vi "4. SJCubeRunExp.vi"() -> ()   [LabVIEW 2019, in "SJCube.lvlib"]
uses:
  SJCube.lvlib
  PendulumState.ctl
  <vilib>/Platform/TimedLoop/XDataNode/timing_clust.ctl
  <vilib>/Platform/TimedLoop/XDataNode/nitl_modes.ctl
  <vilib>/Platform/TimedLoop/XDataNode/wakeup.ctl
  <vilib>/myRIO/Common/Instrument Driver Framework/myRIO v1.0/UART/vis/myRIO v1.0 Close UART.vi
  <vilib>/addons/control/pid/pid.llb/PID (DBL).vi
  <vilib>/myRIO/Common/Instrument Driver Framework/Utilities/vis/FPGA Ref Manager.vi
  <vilib>/myRIO/Common/Instrument Driver Framework/myRIO v1.0/myRIO v1.0 Reset FPGA.vi
  <vilib>/myRIO/Common/Instrument Driver Framework/myRIO v1.0/IRQ/vis/myRIO v1.0 IRQ Info FGV.vi
  <vilib>/myRIO/Common/Instrument Driver Framework/myRIO v1.0/IRQ/vis/myRIO v1.0 Timer IRQ Info FGV.vi
  <vilib>/myRIO/Common/Instrument Driver Framework/myRIO v1.0/IRQ/vis/myRIO v1.0 ISR Agent.vi
  <vilib>/myRIO/Instrument Drivers/Utilities/vis/Reset Index.vi
  <vilib>/myRIO/Common/Instrument Driver Framework/myRIO v1.0/Resource Manager/vis/myRIO v1.0 Block Write Resource Manager.vi
  <vilib>/Platform/TimedLoop/XDataNode/XDataNode.xnode
  <vilib>/Platform/TimedLoop/XDataNode/XDNodeRunTimeDep.lvlib
  <vilib>/myRIO/Instrument Drivers/Utilities/Utilities.lvlib
  <vilib>/addons/control/pid/NI_PID_pid.lvlib
  KNRmBalanceStick-Program/KNRm_ReMi_OS5.lvlibp
  KNRmBalanceStick-Program/KNRm_ReMi_OS5.lvlibp/KNRm_ReMi_Toolkit/IO/LowLevel/IO_Channel_DIO.ctl
panel:
  in  "StickPosControl":bool=TRUE
  out "touch":bool
  in  "Auto\nSetpoint":bool
  out "LATE":bool
  out "停滯":bool
  out "方向":bool
  out "Array":T1[](array[typedef])
  in  "motorPID":T2={"proportional gain (Kc)"=5.0, "integral time (Ti, min)"=0.0, "derivative time (Td, min)"=0.0005}
  in  "PosPID":T2={"proportional gain (Kc)"=-0.05999999999999999, "integral time (Ti, min)"=0.03, "derivative time (Td, min)"=0.019999999999999997}
  in  "BalancePID":T2={"proportional gain (Kc)"=0.07999999999999999, "integral time (Ti, min)"=0.0, "derivative time (Td, min)"=0.0008}
  out "nowState":T1
  out "Waveform Chart":T3(graph)
  in  "Setpoint(deg)":dbl(knob) scale=80.0..-80.0
  out "error out":errorcluster
  out "Position(deg)":dbl(knob) scale=80.0..-80.0
  in  "Reset":bool
  in  "Stop Button":bool
  out "MotorResetPOS":dbl[](array[numeric])
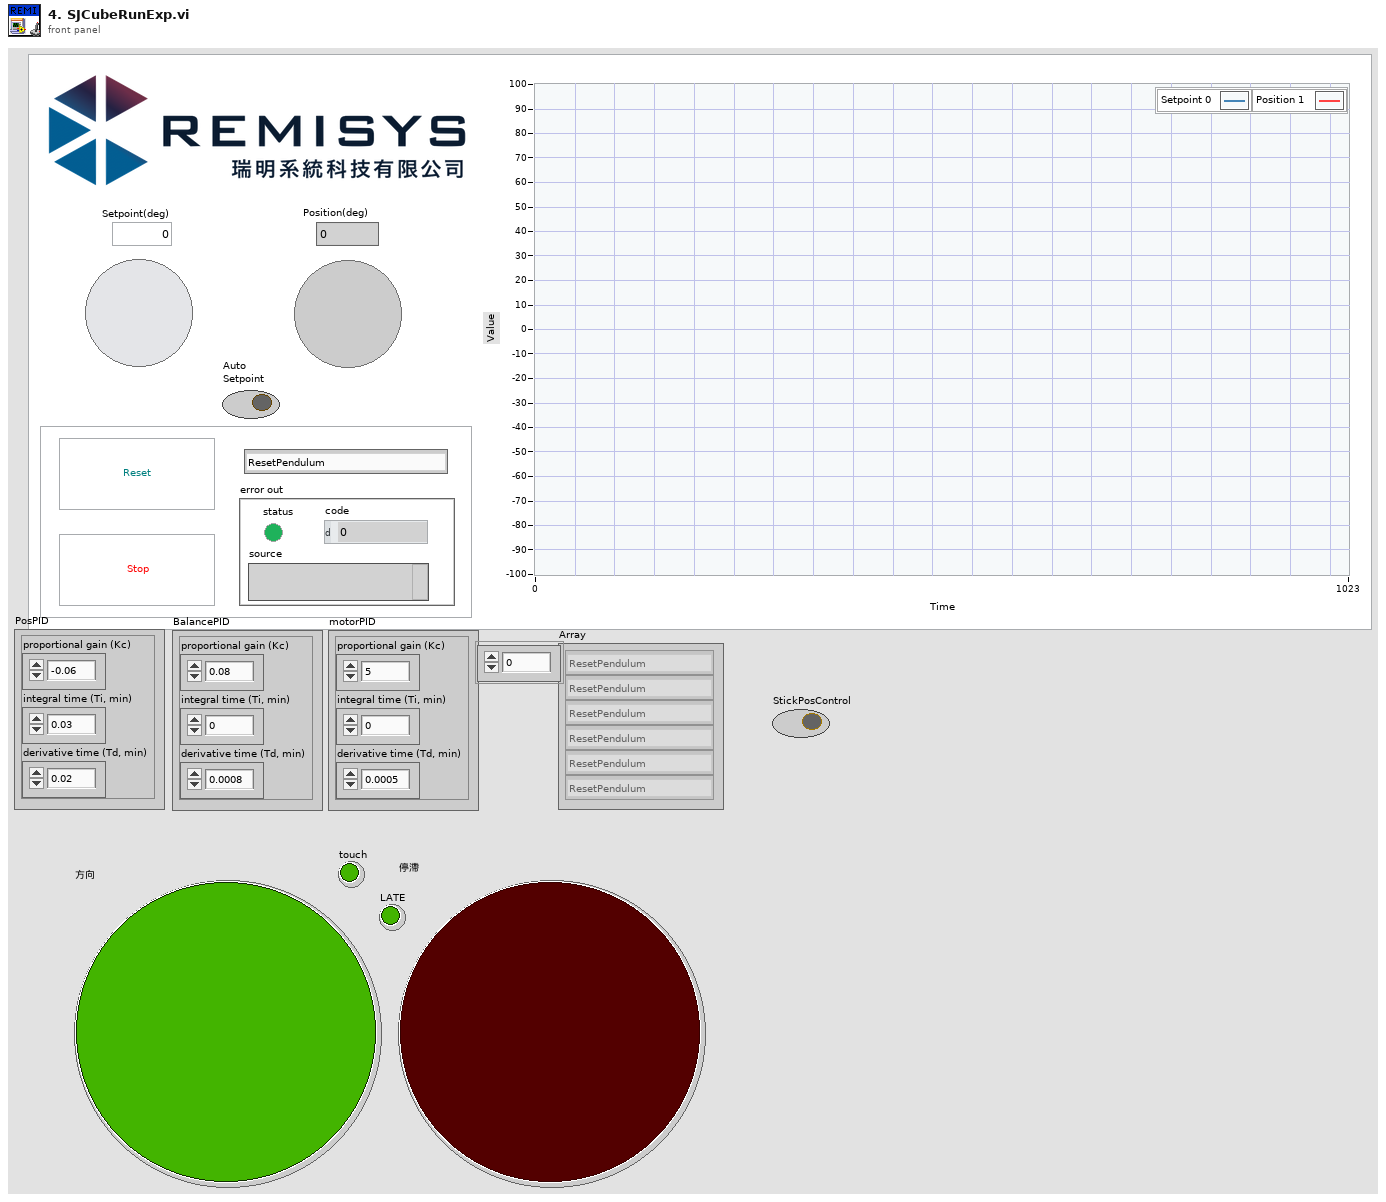
[diagram p1: front panel]
types:
  T1 = typedef "SJCube.lvlib/PendulumState.ctl" = enum16{"ResetPendulum", "PendulumFindHome", "PendulumToHome", "SwingUp", "Balancing", "ExitExp."}
  T2 = cluster{"proportional gain (Kc)":dbl, "integral time (Ti, min)":dbl, "derivative time (Td, min)":dbl}
  T3 = cluster{"Setpoint(deg)":dbl, "PresentPOS(deg)":dbl}
  T4 = typedef "KNRm_ReMi_OS5.lvlibp/IO_Channel_DIO.ctl" = enum16{"B/DIO1 (M1)", "A/DIO8 (M2)", "B/DIO7 (M3)", "A/DIO3 (M4)", "A/DIO14 (RC1_0)", "A/DIO15 (RC1_1)"}
  T5 = typedef "XDNodeRunTimeDep.lvlib/timing_clust.ctl" = cluster{"Expected End [f-1]":u64, "Actual End [f-1]":u64, "Finished Late? [f-1]":bool, "Expected End [i-1]":u64, "Actual End [i-1]":u64, "Finished Late? [i-1]":bool, "Expected Start [i]":u64, "Actual Start [i]":u64, "Expected Start [f]":u64, "Actual Start [f]":u64, "Source Name":string, "Structure Name":string, "Period":i64, "Deadline":i64, "Offset":i64, "Start":i64, "Priority":i32, "Timeout":i32, "Mode":T6, "Wakeup Reason":T7, "Error":errorcluster, "Source Type":string, "Secondary Source Type":string, "Global End Time":u64, "Global Start Time":u64, "Frame Duration":u64, "Iteration Duration":u64, "Assigned CPU":i32, "I/O Scan Engine Mode":u32}
  T6 = typedef "XDNodeRunTimeDep.lvlib/nitl_modes.ctl" = enum32{"No Change", "Process missed periods, maintain original phase", "Discard missed periods, maintain original phase", "Process missed periods, ignore original phase", "Discard missed periods, ignore original phase"}
  T7 = typedef "XDNodeRunTimeDep.lvlib/wakeup.ctl" = enum32{"Normal", "Aborted", "Asynchronous wakeup", "Timing source error", "Timed loop error", "Timeout"}
  T8 = cluster{"Setpoint(deg)":dbl, "MotorEncoder (deg)":dbl}
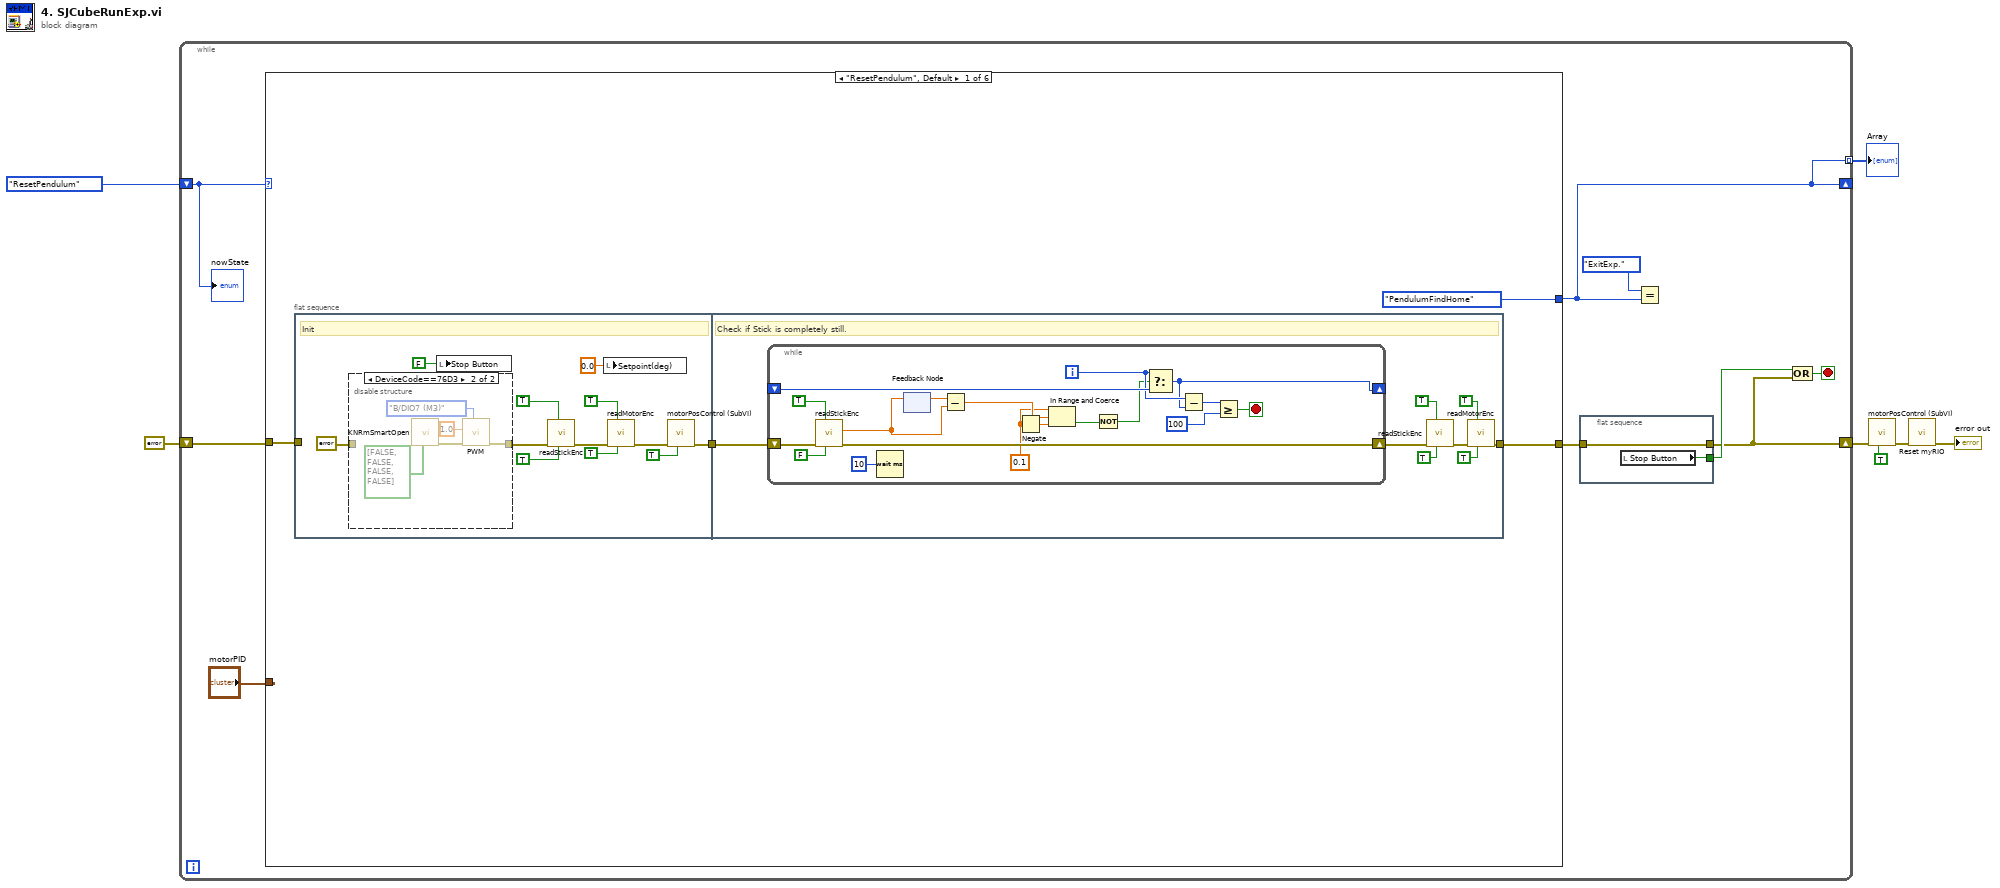
[diagram p0: block diagram]
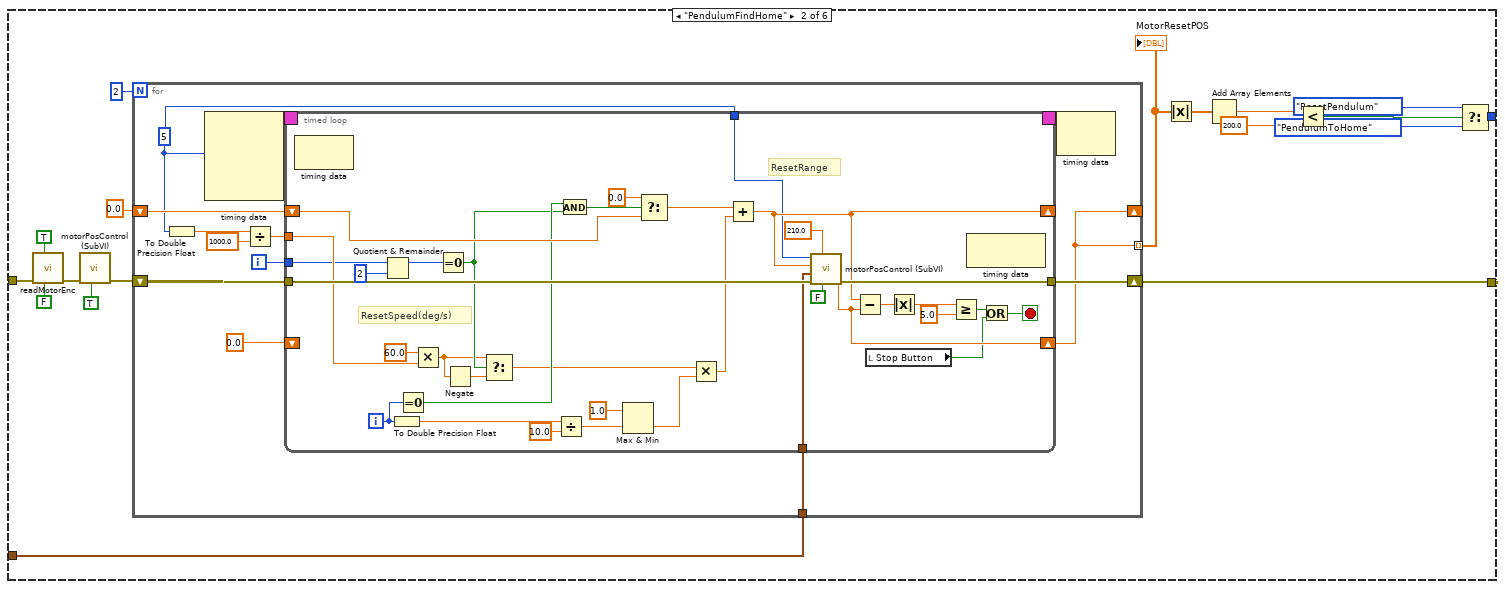
[diagram p3: hidden frame]
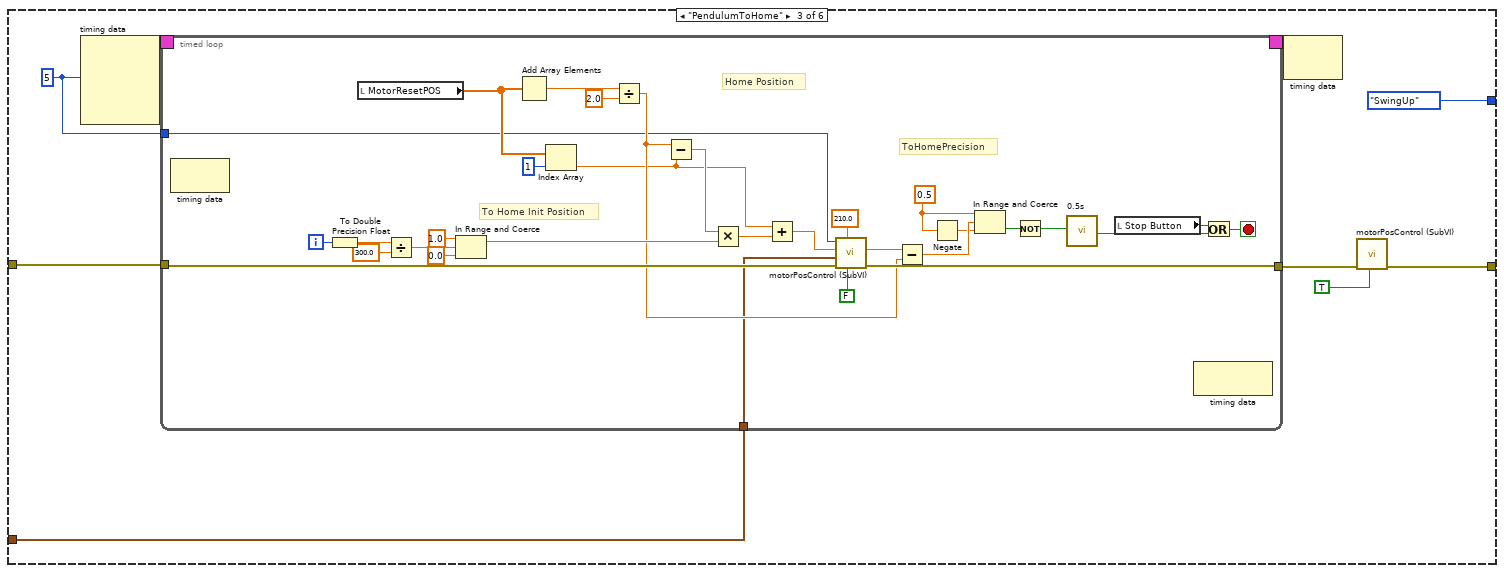
[diagram p4: hidden frame]
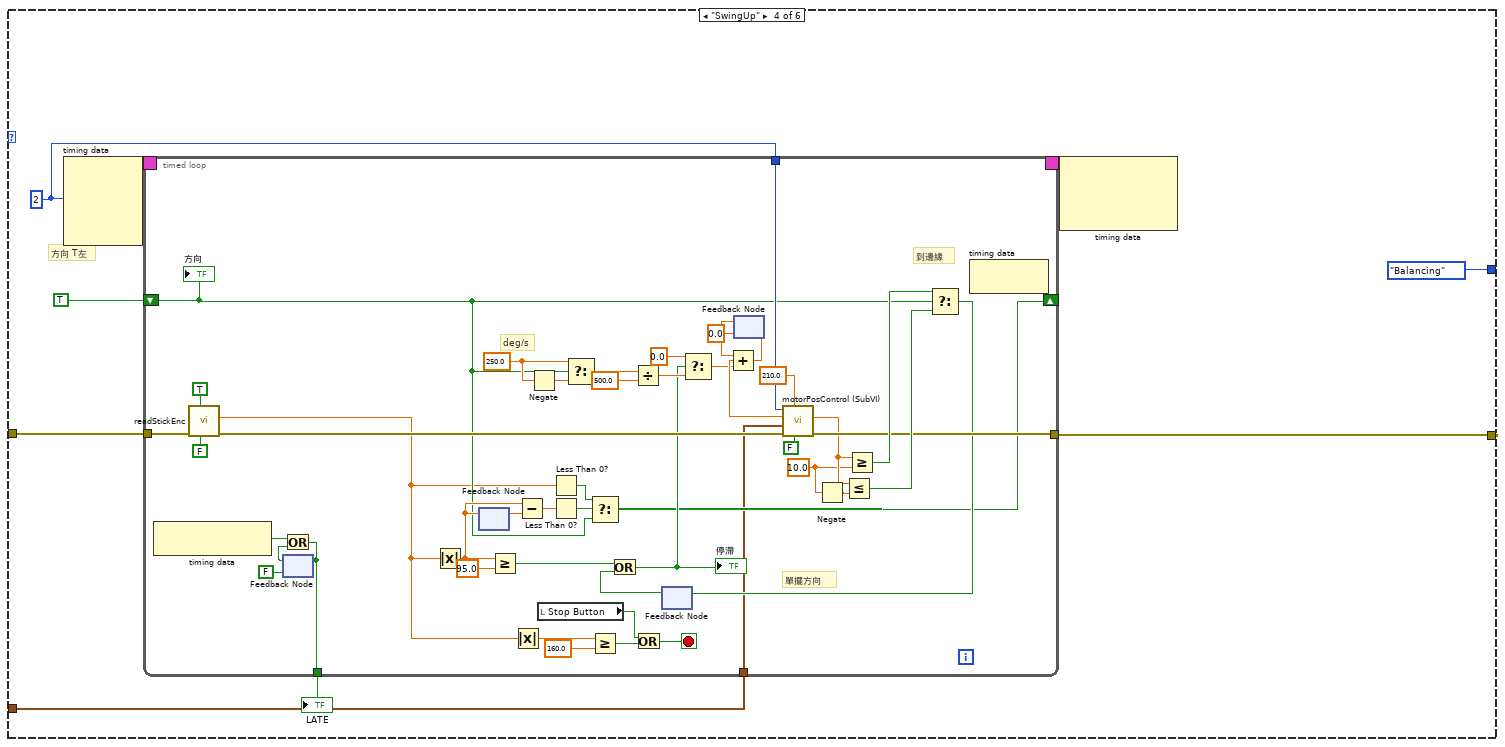
[diagram p5: hidden frame]
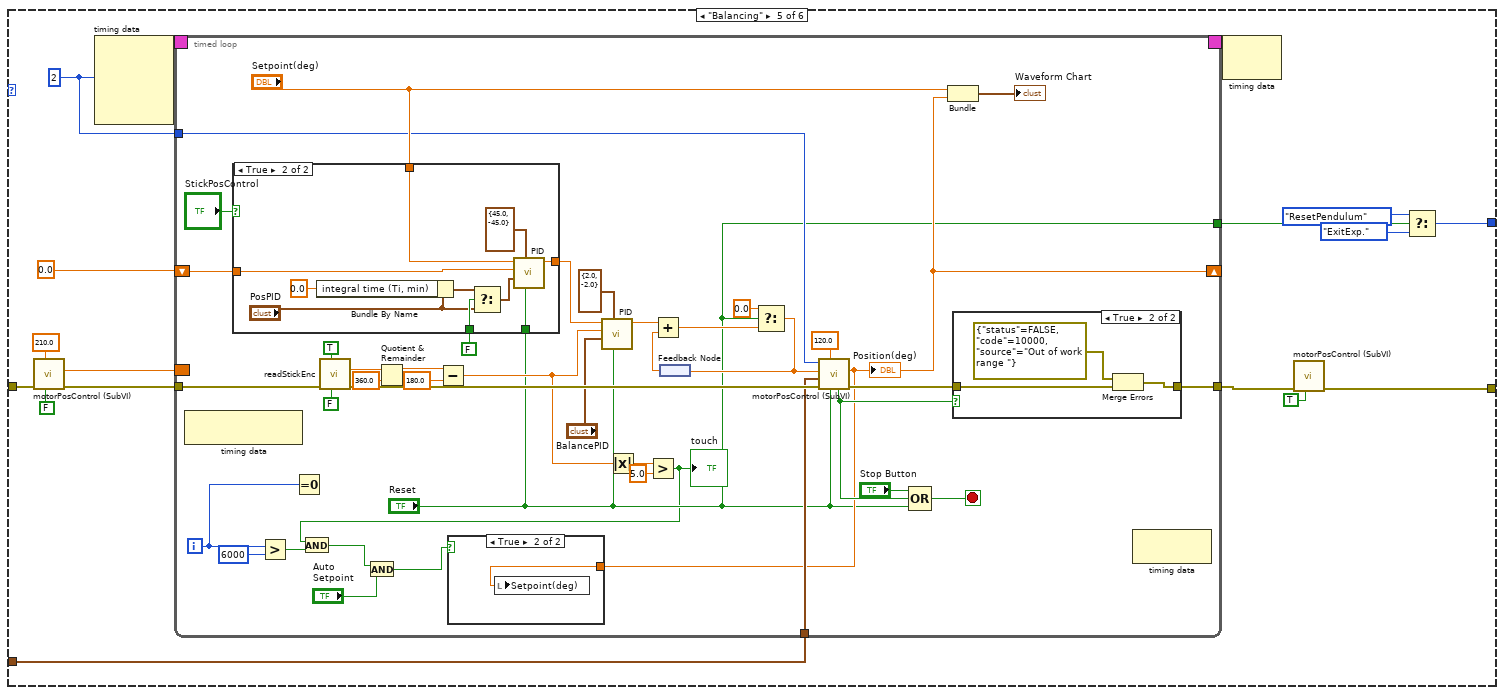
[diagram p6: hidden frame]
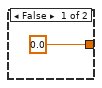
[diagram p8: hidden frame]
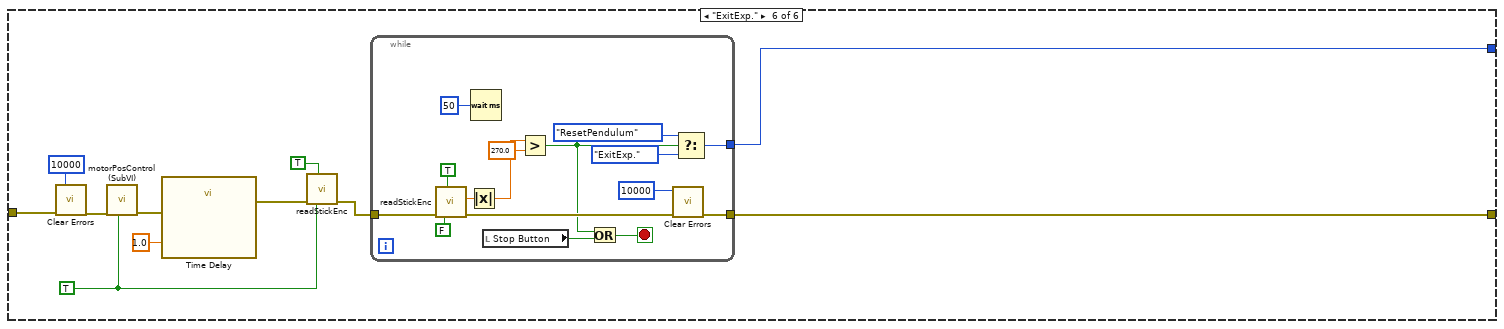
[diagram p10: hidden frame]
diagram:
  n1 = while {
    shift-right: [w8] -> _
    shift-left: PendulumState."ResetPendulum" ("Start State") -> [w13]
    shift-right: [w11] -> w4
    shift-left: errorcluster {"status"=FALSE, "code"=0, "source"=""} ("error in (no error)") -> [w16]
    tunnel: [w8] -> w5 mode=indexing
    stop <- w10 stop-if-true
    n2 = case shown="\"ResetPendulum\", Default" w13 {
      tunnel: w16 -> [w20 w81 w144 w190 w263 w334]
      tunnel: [w21 w84 w141 w189 w260 w333] -> w15
      tunnel: [PendulumState."PendulumFindHome" w70 PendulumState."SwingUp" PendulumState."Balancing" w257 w336] -> w8
      tunnel: "motorPID" -> [_ w69 w139 w185 w248 _]
      frame "ResetPendulum", Default {
        n3 = flat-sequence {
          tunnel: w20 -> [_]
          tunnel: [w27] -> w19
          tunnel: [w44] -> w21
          tunnel: w19 -> [w41]
          frame #0 {
            # "Init"
            n4 = disable-structure shown="DeviceCode==76D3" {
              disable-tunnel: errorcluster {"status"=FALSE, "code"=0, "source"=""} ("error in (no error)") -> [w35 _]
              disable-tunnel: [w35 w37] -> w24
              frame condition #0 (active) {
              }
              frame condition #1 {
                n5 = call "KNRmSmartOpen.vi"("SpeedMode"=bool[] [FALSE, FALSE, FALSE, FALSE]) -> ("error out"=w38:errorcluster)  [unwired: 8 in, 2 out]
                n6 = call "PWM.vi"("IO_Chanel"=IO_Channel_DIO."B/DIO7 (M3)", "error in"=w38, "DutyCycle"=1.0) -> ("error out"=w37:errorcluster)  [unwired: 8 in]
              }
            }
            n7 = local write "Stop Button"(FALSE ("Stop Button")) -> ()
            n8 = call "readStickEnc.vi"("Reset Counter"=TRUE, "Reverse ENC?"=TRUE, "error in (no error)"=w24) -> ("error out"=w31:errorcluster)  [unwired: 7 in, 1 out]
            n9 = local write "Setpoint(deg)"(0.0 ("Setpoint(deg)")) -> ()
            n10 = call "readMotorEnc.vi"("Reset Counter"=TRUE, "Reverse ENC?"=TRUE, "error in (no error)"=w31) -> ("error out"=w28:errorcluster)  [unwired: 7 in, 1 out]
            n11 = call "motorPosControl (SubVI).vi"("Reset"=TRUE, "error in (no error)"=w28) -> ("error out"=w27:errorcluster)  [unwired: 6 in, 3 out]
          }
          frame #1 {
            # "Check if Stick is completely still."
            n12 = while {
              shift-right: [w66] -> w48
              shift-left: w41 -> [w65]
              shift-right: [w54] -> _
              shift-left: _ -> [w56]
              i -> [w55]
              stop <- w51 stop-if-true
              w62 = 0.1 ("upper limit")
              n13 = call "readStickEnc.vi"("Reset Counter"=FALSE, "Reverse ENC?"=TRUE, "error in (no error)"=w65) -> ("error out"=w66:errorcluster, "StickEncoder (deg)"=w60:dbl)  [unwired: 7 in]
              n14 = Wait (ms)(milliseconds to wait=u32 10) -> ()  [unwired: 1 out]
              n15 = feedback-in #1(w60) -> ()
              n16 = feedback #1() -> (w64:dbl)  [unwired: 1 in]
              n17 = Subtract(x=w64, y=w60) -> (x-y=w63:dbl)
              n18 = Negate(x=w62) -> (-x=w61:dbl)
              n19 = In Range and Coerce(upper limit=w62, x=w63, lower limit=w61) -> (In Range?=w50:bool)  [unwired: 1 out]
              n20 = Not(x=w50) -> (.not. x?=w49:bool)
              n21 = Select(t=w55, s=w49, f=w56) -> (s? t:f=w54:i32)
              n22 = Subtract(x=w55, y=w54) -> (x-y=w53:i32)
              n23 = Greater Or Equal?(x=w53, y=100) -> (x >= y?=w51:bool)
            }
            n24 = call "readStickEnc.vi"("Reset Counter"=TRUE, "Reverse ENC?"=TRUE, "error in (no error)"=w48) -> ("error out"=w45:errorcluster)  [unwired: 7 in, 1 out]
            n25 = call "readMotorEnc.vi"("Reset Counter"=TRUE, "Reverse ENC?"=TRUE, "error in (no error)"=w45) -> ("error out"=w44:errorcluster)  [unwired: 7 in, 1 out]
          }
        }
      }
      frame "PendulumFindHome" {
        n26 = call "readMotorEnc.vi"("Reset Counter"=FALSE, "Reverse ENC?"=TRUE ("Reset Button"), "error in (no error)"=w81) -> ("error out"=w82:errorcluster)  [unwired: 7 in, 1 out]
        n27 = call "motorPosControl (SubVI).vi"("Reset"=TRUE, "error in (no error)"=w82) -> ("error out"=w77:errorcluster)  [unwired: 6 in, 3 out]
        n28 = for {
          N: 2 -> [_]
          shift-right: [w95] -> w84
          shift-left: w77 -> [w94]
          shift-right: [w88] -> _
          shift-left: 0.0 ("PresentPOS(deg)") -> [w92]
          tunnel: [w88] -> w68 mode=indexing
          tunnel: w69 -> [w86]
          i -> [w93]
          w85 = i64 5 ("Period")
          n29 = To Double Precision Float(number=w85) -> (double precision float=w91:dbl)
          n30 = node-c288(w85) -> (w97:T5)  [unwired: 3 in]
          n31 = Divide(x=w91, y=1000.0) -> (x/y=w89:dbl)
          n32 = timed-loop {
            timing: w97 -> [_]
            timing-out: [_] -> w96
            tunnel: w94 -> [w127]
            tunnel: [w126] -> w95
            tunnel: w93 -> [w111]
            shift-right: [w122] -> _
            shift-left: w92 -> [w110]
            tunnel: w89 -> [w118]
            shift-right: [w117] -> w88
            shift-left: 0.0 ("MotorEncoder (deg)") -> [_]
            tunnel: w86 -> [w99]
            tunnel: w85 -> [w98]
            i -> [w106]
            stop <- w131 stop-if-true
            # "ResetRange"
            # "ResetSpeed(deg/s)"
            n33 = node-c288() -> ()  [unwired: 1 in, 1 out]
            n34 = Quotient & Remainder(x=w111, y=2) -> (x-y*floor(x/y)=w107:i32)  [unwired: 1 out]
            n35 = To Double Precision Float(number=w106) -> (double precision float=w123:dbl)
            n36 = Equal To 0?(x=w106) -> (x = 0?=w104:bool)
            n37 = Multiply(x=60.0 ("y"), y=w118) -> (x*y=w102:dbl)
            n38 = Equal To 0?(x=w107) -> (x = 0?=w103:bool)
            n39 = Negate(x=w102) -> (-x=w101:dbl)
            n40 = Select(t=w102, s=w103, f=w101) -> (s? t:f=w100:dbl)
            n41 = Divide(x=w123, y=10.0) -> (x/y=w121:dbl)
            n42 = And(x=w104, y=w103) -> (x .and. y?=w105:bool)
            n43 = Max & Min(x=1.0 ("upper limit"), y=w121) -> (min(x,y)=w116:dbl)  [unwired: 1 out]
            n44 = Select(t=0.0, s=w105, f=w110) -> (s? t:f=w108:dbl)
            n45 = Multiply(x=w100, y=w116) -> (x*y=w113:dbl)
            n46 = Add(x=w108, y=w113) -> (x+y=w122:dbl)
            n47 = call "motorPosControl (SubVI).vi"("Reset"=FALSE, "+/- Range"=210.0 ("WorkRange"), "error in (no error)"=w127, "PID gains"=w99, "Position (deg)"=w122, "dt"=w98) -> ("error out"=w126:errorcluster, "MotorEncoder (deg)"=w117:dbl)  [unwired: 2 in, 2 out]
            n48 = Subtract(x=w122, y=w117) -> (x-y=w129:dbl)
            n49 = local read "Stop Button"() -> (w114:bool)
            n50 = Absolute Value(x=w129) -> (abs(x)=w128:dbl)
            n51 = Greater Or Equal?(x=w128, y=5.0) -> (x >= y?=w115:bool)
            n52 = node-c288() -> ()  [unwired: 1 in, 1 out]
            n53 = Or(x=w115, y=w114) -> (x .or. y?=w131:bool)
          }
          n54 = node-c288(w96) -> ()  [unwired: 1 out]
        }
        "MotorResetPOS" <- w68
        n55 = Absolute Value(x=w68) -> (abs(x)=w67:dbl[])
        n56 = Add Array Elements(numeric array=w67) -> (sum=w75:dbl)
        n57 = Less?(x=w75, y=200.0) -> (x < y?=w73:bool)
        n58 = Select(t=PendulumState."ResetPendulum", s=w73, f=PendulumState."PendulumToHome") -> (s? t:f=w70:T1)
      }
      frame "PendulumToHome" {
        w140 = i64 5 ("Period")
        n59 = node-c288(w140) -> (w146:T5)  [unwired: 3 in]
        n60 = timed-loop {
          timing: w146 -> [_]
          timing-out: [_] -> w145
          tunnel: w144 -> [w178]
          tunnel: [w173] -> w143
          tunnel: w140 -> [w149]
          tunnel: w139 -> [w148]
          i -> [w172]
          stop <- w158 stop-if-true
          w175 = 0.5
          # "To Home Init Position"
          # "Home Position"
          # "ToHomePrecision"
          n61 = node-c288() -> ()  [unwired: 1 in, 1 out]
          n62 = To Double Precision Float(number=w172) -> (double precision float=w155:dbl)
          n63 = local read "MotorResetPOS"() -> (w167:dbl[])
          n64 = Divide(x=w155, y=300.0) -> (x/y=w170:dbl)
          n65 = In Range and Coerce(upper limit=1.0, x=w170, lower limit=0.0) -> (coerced(x)=w165:dbl)  [unwired: 1 out]
          n66 = Add Array Elements(numeric array=w167) -> (sum=w166:dbl)
          n67 = Index Array(array=w167, index=1) -> (element=w161:dbl)
          n68 = Divide(x=w166, y=2.0) -> (x/y=w163:dbl)
          n69 = Subtract(x=w163, y=w161) -> (x-y=w162:dbl)
          n70 = Multiply(x=w162, y=w165) -> (x*y=w164:dbl)
          n71 = Add(x=w161, y=w164) -> (x+y=w160:dbl)
          n72 = call "motorPosControl (SubVI).vi"("Reset"=FALSE, "+/- Range"=210.0 ("WorkRange"), "error in (no error)"=w178, "PID gains"=w148, "Position (deg)"=w160, "dt"=w149) -> ("error out"=w173:errorcluster, "MotorEncoder (deg)"=w177:dbl)  [unwired: 2 in, 2 out]
          n73 = Subtract(x=w177, y=w163) -> (x-y=w176:dbl)
          n74 = Negate(x=w175) -> (-x=w174:dbl)
          n75 = In Range and Coerce(upper limit=w175, x=w176, lower limit=w174) -> (In Range?=w154:bool)  [unwired: 1 out]
          n76 = Not(x=w154) -> (.not. x?=w153:bool)
          n77 = call "0.5s"("Reset"=w153) -> ("Time has Elapsed"=w151:bool)  [unwired: 11 in, 7 out]
          n78 = local read "Stop Button"() -> (w150:bool)
          n79 = node-c288() -> ()  [unwired: 1 in, 1 out]
          n80 = Or(x=w150, y=w151) -> (x .or. y?=w158:bool)
        }
        n81 = node-c288(w145) -> ()  [unwired: 1 out]
        n82 = call "motorPosControl (SubVI).vi"("Reset"=TRUE ("Reset Button"), "error in (no error)"=w143) -> ("error out"=w141:errorcluster)  [unwired: 6 in, 3 out]
      }
      frame "SwingUp" {
        w188 = i64 2 ("Period")
        # "方向 T左"
        n83 = node-c288(w188) -> (w192:T5)  [unwired: 3 in]
        n84 = timed-loop {
          timing: w192 -> [_]
          timing-out: [_] -> w191
          tunnel: w190 -> [w231]
          tunnel: [w230] -> w189
          tunnel: w188 -> [w223]
          shift-right: [w202] -> _
          shift-left: TRUE -> [w206]
          tunnel: [w198] -> w186
          tunnel: w185 -> [w195]
          stop <- w237 stop-if-true
          w197 = 10.0 ("UpLimit")
          w216 = 250.0
          # "deg/s"
          # "單擺方向"
          # "到邊緣"
          n85 = node-c288() -> (w201:bool)  [unwired: 1 in]
          n86 = call "readStickEnc.vi"("Reset Counter"=FALSE, "Reverse ENC?"=TRUE, "error in (no error)"=w231) -> ("error out"=w228:errorcluster, "StickEncoder (deg)"=w194:dbl)  [unwired: 7 in]
          n87 = feedback #2(FALSE) -> (w200:bool)
          n88 = Or(x=w201, y=w200) -> (x .or. y?=w198:bool)
          n89 = feedback-in #2(w198) -> ()
          n90 = Absolute Value(x=w194) -> (abs(x)=w208:dbl)
          n91 = feedback-in #3(w208) -> ()
          n92 = feedback #3() -> (w214:dbl)  [unwired: 1 in]
          n93 = Greater Or Equal?(x=w208, y=95.0) -> (x >= y?=w211:bool)
          n94 = Absolute Value(x=w194) -> (abs(x)=w239:dbl)
          n95 = Subtract(x=w208, y=w214) -> (x-y=w213:dbl)
          n96 = Negate(x=w216) -> (-x=w217:dbl)
          n97 = local read "Stop Button"() -> (w227:bool)
          n98 = Less Than 0?(x=w194) -> (x < 0?=w205:bool)
          n99 = Less Than 0?(x=w213) -> (x < 0?=w207:bool)
          n100 = Select(t=w216, s=w206, f=w217) -> (s? t:f=w218:dbl)
          n101 = Select(t=w205, s=w207, f=w206) -> (s? t:f=w202:bool)
          n102 = Greater Or Equal?(x=w239, y=160.0) -> (x >= y?=w204:bool)
          n103 = Divide(x=w218, y=500.0 ("x")) -> (x/y=w220:dbl)
          n104 = Or(x=w227, y=w204) -> (x .or. y?=w237:bool)
          n105 = feedback #4() -> (w209:bool)  [unwired: 1 in]
          n106 = Or(x=w211, y=w209) -> (x .or. y?=w212:bool)
          "停滯" <- w212
          n107 = Select(t=0.0, s=w212, f=w220) -> (s? t:f=w219:dbl)
          n108 = feedback #5(0.0) -> (w236:dbl)
          n109 = Add(x=w236, y=w219) -> (x+y=w226:dbl)
          n110 = feedback-in #5(w226) -> ()
          n111 = call "motorPosControl (SubVI).vi"("Reset"=FALSE, "+/- Range"=210.0 ("WorkRange"), "error in (no error)"=w228, "PID gains"=w195, "Position (deg)"=w226, "dt"=w223) -> ("error out"=w230:errorcluster, "MotorEncoder (deg)"=w203:dbl)  [unwired: 2 in, 2 out]
          n112 = Negate(x=w197) -> (-x=w196:dbl)
          n113 = Less Or Equal?(x=w203, y=w196) -> (x <= y?=w233:bool)
          n114 = Greater Or Equal?(x=w203, y=w197) -> (x >= y?=w234:bool)
          n115 = Select(t=w234, s=w206, f=w233) -> (s? t:f=w210:bool)
          n116 = feedback-in #4(w210) -> ()
          n117 = node-c288() -> ()  [unwired: 1 in, 1 out]
          "方向" <- w206
        }
        "LATE" <- w186
        n118 = node-c288(w191) -> ()  [unwired: 3 out]
      }
      frame "Balancing" {
        w247 = i64 2 ("Period")
        n119 = call "motorPosControl (SubVI).vi"("Reset"=FALSE ("Reset Button"), "+/- Range"=210.0, "error in (no error)"=w263) -> ("error out"=w253:errorcluster, "MotorEncoder (deg)"=w252:dbl)  [unwired: 5 in, 2 out]
        n120 = node-c288(w247) -> (w256:T5)  [unwired: 3 in]
        n121 = timed-loop "Timed Loop" {
          timing: w256 -> [_]
          timing-out: [_] -> w255
          border: w252 -> [_]
          shift-right: [w272] -> _
          shift-left: 0.0 -> [w283]
          tunnel: w253 -> [w289]
          tunnel: ["Reset"] -> w251
          tunnel: [w287] -> w250
          tunnel: w247 -> [w281]
          tunnel: w248 -> [w280]
          i -> [w267]
          stop <- w298 stop-if-true
          n122 = node-c288() -> ()  [unwired: 1 in, 1 out]
          n123 = case shown="True" "StickPosControl" {
            tunnel: [0.0 ("output") w315] -> w275
            tunnel: w283 -> [_ w314]
            tunnel: "Reset" -> [_ w313]
            tunnel: "Setpoint(deg)" -> [_ w312]
            tunnel: FALSE -> [_ w311]
            frame False {
            }
            frame True {
              n124 = Bundle By Name(cluster="PosPID", "integral time (Ti, min)"=0.0) -> (w308:T2)
              n125 = Select(t=w308, s=w311, f="PosPID") -> (s? t:f=w310:T2)
              n126 = call-poly <vilib>:"PID.vi"("reinitialize? (F)"=w313, "output range"=cluster{"output high":dbl, "output low":dbl} {"output high"=45.0, "output low"=-45.0}, "PID gains"=w310, "process variable"=w314, "setpoint"=w312) -> ("output"=w315:dbl)  [unwired: 5 in, 1 out]
            }
          }
          n127 = Greater?(x=w267, y=6000) -> (0:w276:bool)
          n128 = Equal To 0?(x=w267) -> ()  [unwired: 1 out]
          n129 = call "readStickEnc.vi"("Reset Counter"=FALSE, "Reverse ENC?"=TRUE, "error in (no error)"=w289) -> ("error out"=w291:errorcluster, "StickEncoder (deg)"=w292:dbl)  [unwired: 7 in]
          n130 = Quotient & Remainder(x=w292, y=360.0) -> (x-y*floor(x/y)=w299:dbl)  [unwired: 1 out]
          n131 = Subtract(x=w299, y=180.0) -> (x-y=w271:dbl)
          n132 = call-poly <vilib>:"PID.vi"("reinitialize? (F)"="Reset", "output range"=cluster{"output high":dbl, "output low":dbl} {"output high"=2.0, "output low"=-2.0}, "PID gains"="BalancePID", "process variable"=w271, "setpoint"=w275) -> ("output"=w279:dbl)  [unwired: 5 in, 1 out]
          n133 = Absolute Value(x=w271) -> (abs(x)=w274:dbl)
          n134 = Greater?(x=w274, y=5.0) -> (0:w265:bool)
          "touch" <- w265
          n135 = And(x=w265, y=w276) -> (x .and. y?=w270:bool)
          n136 = And(x=w270, y="Auto\nSetpoint") -> (x .and. y?=w268:bool)
          n137 = feedback #6() -> (w278:dbl)
          n138 = Add(x=w279, y=w278) -> (x+y=w303:dbl)
          n139 = Select(t=0.0, s="Reset", f=w303) -> (s? t:f=w293:dbl)
          n140 = feedback-in #6(w293) -> ()
          n141 = call "motorPosControl (SubVI).vi"("Reset"="Reset", "+/- Range"=120.0 ("WorkRange"), "error in (no error)"=w291, "PID gains"=w280, "Position (deg)"=w293, "dt"=w281) -> ("error out"=w295:errorcluster, "MotorEncoder (deg)"=w272:dbl, "out of range!"=w296:bool)  [unwired: 2 in, 1 out]
          "Position(deg)" <- w272
          n142 = case shown="True" w268 {
            tunnel: w272 -> [_ w305]
            frame False {
            }
            frame True {
              n143 = local write "Setpoint(deg)"(w305) -> ()
            }
          }
          n144 = Compound Arithmetic op=OR("Stop Button", w296, "Reset") -> (w298:bool)
          n145 = Bundle("Setpoint(deg)"="Setpoint(deg)", "MotorEncoder (deg)"=w272) -> (→"Waveform Chart":T8)  [unwired: 1 in]
          n146 = case shown="True" w296 {
            tunnel: w295 -> [w317 w320]
            tunnel: [w317 w318] -> w287
            frame False {
            }
            frame True {
              n147 = Merge Errors(errorcluster {"status"=FALSE, "code"=10000, "source"="Out of work range "} ("error in (no error)"), w320) -> (w318:errorcluster)
            }
          }
          n148 = node-c288() -> ()  [unwired: 1 in, 1 out]
        }
        n149 = node-c288(w255) -> ()  [unwired: 1 out]
        n150 = call "motorPosControl (SubVI).vi"("Reset"=TRUE ("Reset Button"), "error in (no error)"=w250) -> ("error out"=w260:errorcluster)  [unwired: 6 in, 3 out]
        n151 = Select(t=PendulumState."ResetPendulum", s=w251, f=PendulumState."ExitExp.") -> (s? t:f=w257:T1)
      }
      frame "ExitExp." {
        w330 = TRUE ("Reset Counter")
        n152 = call <vilib>:"Clear Errors.vi"("error in (no error)"=w334, "specific error code to clear (0: all)"=10000) -> ("error out"=w332:errorcluster)  [unwired: 4 in, 1 out]
        n153 = call "motorPosControl (SubVI).vi"("Reset"=w330, "error in (no error)"=w332) -> ("error out"=w331:errorcluster)  [unwired: 6 in, 3 out]
        n154 = call "Time Delay"("error in (no error)"=w331, "Delay Time (s)"=1.0) -> ("error out"=w329:errorcluster)  [unwired: 9 in]
        n155 = call "readStickEnc.vi"("Reset Counter"=w330, "Reverse ENC?"=TRUE, "error in (no error)"=w329) -> ("error out"=w327:errorcluster)  [unwired: 7 in, 1 out]
        n156 = while {
          tunnel: w327 -> [w353]
          tunnel: [w347] -> w336
          tunnel: [w343] -> w333
          stop <- w340 stop-if-true
          n157 = call "readStickEnc.vi"("Reset Counter"=FALSE, "Reverse ENC?"=TRUE, "error in (no error)"=w353) -> ("error out"=w344:errorcluster, "StickEncoder (deg)"=w350:dbl)  [unwired: 7 in]
          n158 = Absolute Value(x=w350) -> (abs(x)=w342:dbl)
          n159 = Wait (ms)(milliseconds to wait=u32 50) -> ()  [unwired: 1 out]
          n160 = local read "Stop Button"() -> (w339:bool)
          n161 = Greater?(x=w342, y=270.0) -> (0:w338:bool)
          n162 = Or(x=w338, y=w339) -> (x .or. y?=w340:bool)
          n163 = call <vilib>:"Clear Errors.vi"("error in (no error)"=w344, "specific error code to clear (0: all)"=10000) -> ("error out"=w343:errorcluster)  [unwired: 4 in, 1 out]
          n164 = Select(t=PendulumState."ResetPendulum", s=w338, f=PendulumState."ExitExp.") -> (s? t:f=w347:T1)
        }
      }
    }
    n165 = flat-sequence {
      tunnel: w15 -> [w17]
      tunnel: [w18] -> w14
      tunnel: [w17] -> w11
      frame #0 {
        n166 = local read "Stop Button"() -> (w18:bool)
      }
    }
    n167 = Equal?(x=PendulumState."ExitExp." ("y"), y=w8) -> ()  [unwired: 1 out]
    n168 = Compound Arithmetic op=OR(w14, w11) -> (w10:bool)
    "nowState" <- w13
  }
  "Array" <- w5
  n169 = call "motorPosControl (SubVI).vi"("Reset"=TRUE, "error in (no error)"=w4) -> ("error out"=w3:errorcluster)  [unwired: 6 in, 3 out]
  n170 = call <vilib>:"Reset myRIO.vi"("error in (no error)"=w3) -> ("error out"=→"error out":errorcluster)  [unwired: 10 in]
